vi "VerticalSpeedIndicator.vi"(6 "SignalSource":T1(ring), 7 "ScaleUnit(F=m/s; T=Ft/min/100)":bool=TRUE, 8 "error in (no error)":errorcluster caption="Fehler (Eingang, kein Fehler)", 10 "MultiWii Data Cluster":T2 {"Altitude abs [m]" format="%.2f"; "Baro T [°C]" format="%.1f"; "Baro P [mbara]" format="%.1f"; "GPS_coord[LON]" format="%#_9f"; "GPS_coord[LAT]" format="%#_9f"; "Altitude [m]" format="%.2f"}) -> (0 "error out":errorcluster caption="Fehler (Ausgang)", 2 "VerticalSpeedDigital":dbl format="%.1f", 3 "VerticalSpeedIndicator":picture)   [LabVIEW 2017]
uses:
  IMU_Functions/IMU_Data_Cluster.ctl
  <vilib>/picture/picture.llb/imagedata.ctl
  <vilib>/Utility/miscctls.llb/LVBoundsTypeDef.ctl
panel:
  in  "Transparent":picture caption="Neue Grafik"
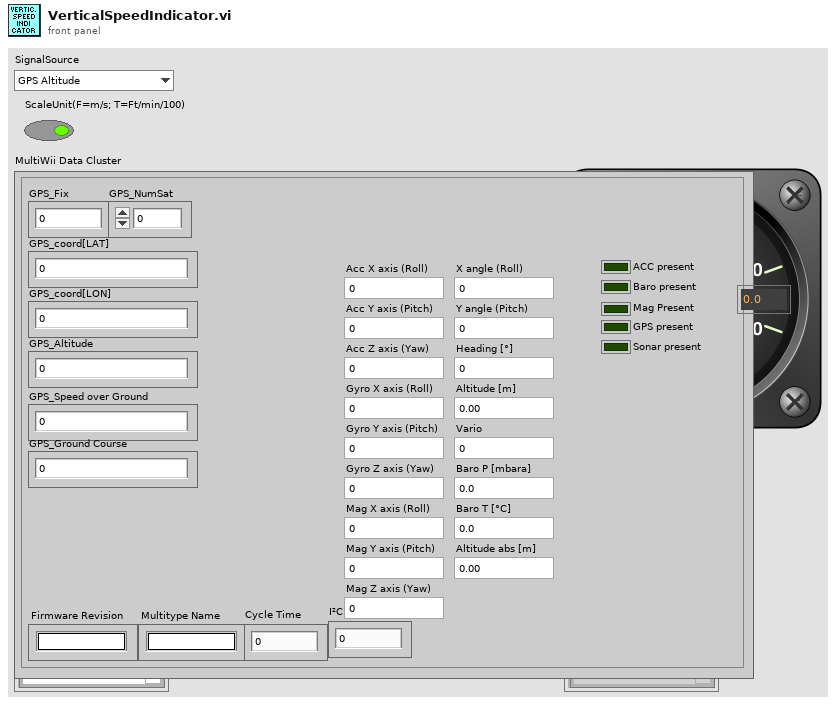
[diagram p1: front panel]
types:
  T1 = enum16{"GPS Altitude", "Baro absolute Altitude", "Baro Vario"}
  T2 = typedef "IMU_Data_Cluster.ctl" = cluster{"Firmware Revision":string, "Multitype Name":string, "Cycle Time":u16, "I²C Error Count":u16, "ACC present":bool, "Baro present":bool, "Mag Present":bool, "GPS present":bool, "Sonar present":bool, "Acc X axis (Roll)":dbl, "Acc Y axis (Pitch)":dbl, "Acc Z axis (Yaw)":dbl, "Gyro X axis (Roll)":dbl, "Gyro Y axis (Pitch)":dbl, "Gyro Z axis (Yaw)":dbl, "Mag X axis (Roll)":dbl, "Mag Y axis (Pitch)":dbl, "Mag Z axis (Yaw)":dbl, "X angle (Roll)":dbl, "Y angle (Pitch)":dbl, "Heading [°]":dbl, "Altitude [m]":dbl, "Vario":dbl, "GPS_Fix":u8, "GPS_NumSat":u8, "GPS_coord[LAT]":dbl, "GPS_coord[LON]":dbl, "GPS_Altitude":dbl, "GPS_Speed over Ground":dbl, "GPS_Ground Course":dbl, "Baro P [mbara]":dbl, "Baro T [°C]":dbl, "Altitude abs [m]":dbl}
  T3 = typedef "LVBoundsTypeDef.ctl" = cluster{"Width":u32, "Height":u32}
  T4 = typedef "imagedata.ctl" = cluster{"image type":i32, "image depth":i32, "image":u8[], "mask":u8[], "colors":u32[], "Rectangle":cluster{"left":i16, "top":i16, "right":i16, "bottom":i16}}
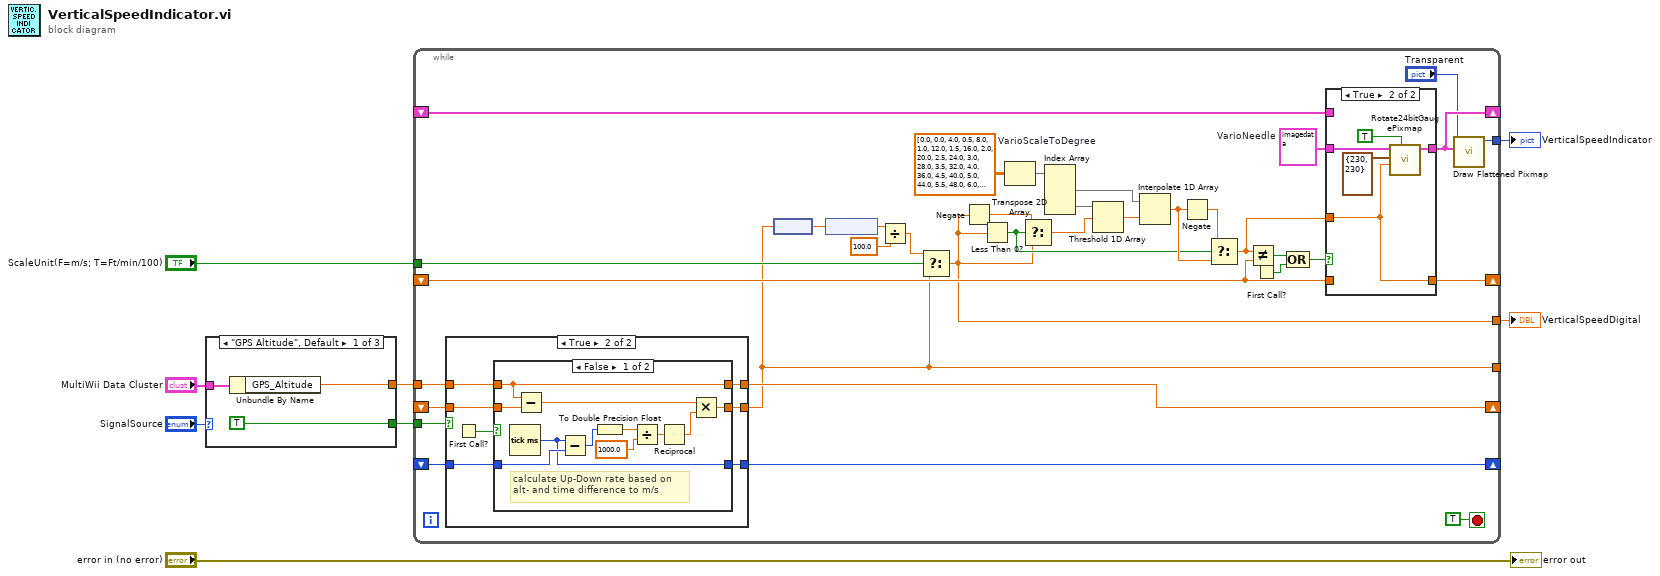
[diagram p0: block diagram]
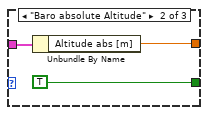
[diagram p2: hidden frame]
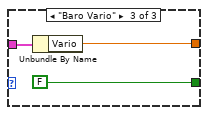
[diagram p3: hidden frame]
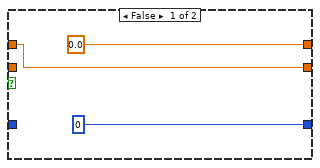
[diagram p4: hidden frame]
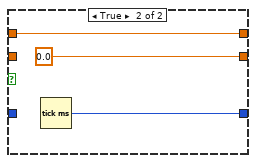
[diagram p5: hidden frame]
diagram:
  n1 = case shown="\"GPS Altitude\", Default" "SignalSource" {
    tunnel: [TRUE TRUE FALSE] -> w2
    tunnel: "MultiWii Data Cluster" -> [w11 w14 w16]
    tunnel: [w10 w12 w15] -> w3
    frame "GPS Altitude", Default {
      n2 = Unbundle By Name(w11) -> ("GPS_Altitude"=w10:dbl)
    }
    frame "Baro absolute Altitude" {
      n3 = Unbundle By Name(w14) -> ("Altitude abs [m]"=w12:dbl)
    }
    frame "Baro Vario" {
      n4 = Unbundle By Name(w16) -> ("Vario"=w15:dbl)
    }
  }
  n5 = while {
    shift-right: [w50] -> _
    shift-left: _ -> [w44]
    shift-right: [w49] -> _
    shift-left: _ -> [w48]
    tunnel: [w46] -> w8
    tunnel: w3 -> [w23]
    tunnel: "ScaleUnit(F=m/s; T=Ft/min/100)" -> [w31]
    tunnel: [w18] -> w1
    tunnel: [w22] -> _
    shift-right: [w26] -> _
    shift-left: _ -> [w27]
    tunnel: w2 -> [w24]
    shift-right: [w21] -> _
    shift-left: _ -> [w20]
    stop <- TRUE stop-if-true
    w42 = dbl[][] [[0.0, 0.0], [4.0, 0.5], [8.0, 1.0], [12.0, 1.5], [16.0, 2.0], [20.0, 2.5], [24.0, 3.0], [28.0, 3.5], [32.0, 4.0], [36.0, 4.5], [40.0, 5.0], [44.0, 5.5], [48.0, 6.0], [52.0, 6.5], [56.0, 7.0], [60.0, 7.5], [64.0, 8.0], [68.0, 8.5], [72.0, 9.0], [76.0, 9.5], [80.0, 10.0], [88.0, 11.0], [96.0, 12.0], [104.0, 13.0], [112.0, 14.0], [120.0, 15.0], [128.0, 16.0], [136.0, 17.0], [144.0, 18.0], [152.0, 19.0], [160.0, 20.0]]  # VarioScaleToDegree
    w43 = T4 {"image type"=0, "image depth"=24, "image"=array[158700 elements], "mask"=[], "colors"=[], "Rectangle"={"left"=0, "top"=0, "right"=230, "bottom"=230}}  # VarioNeedle
    n6 = case shown="True" w24 {
      tunnel: w27 -> [_ w62]
      tunnel: [0.0 ("VerticalSpeed (m/s)") w61] -> w26
      tunnel: w23 -> [w54 w60]
      tunnel: [w54 w58] -> w22
      tunnel: [u32 0 ("millisecond timer value") w57] -> w21
      tunnel: w20 -> [_ w56]
      frame False {
      }
      frame True {
        n7 = First Call?() -> (First Call?: T/F=w59:bool)
        n8 = case shown="False" w59 {
          tunnel: w60 -> [w72 w76]
          tunnel: [w72 w76] -> w61
          tunnel: w62 -> [w73 _]
          tunnel: [w65 0.0] -> w58
          tunnel: [w70 w74] -> w57
          tunnel: w56 -> [w71 _]
          frame False {
            # "calculate Up-Down rate based on\nalt- and time difference to m/s"
            n9 = Tick Count (ms)() -> (millisecond timer value=w70:u32)
            n10 = Subtract(x=w72, y=w73) -> (x-y=w64:dbl)
            n11 = Subtract(x=w70, y=w71) -> (x-y=w69:u32)
            n12 = To Double Precision Float(number=w69) -> (double precision float=w68:dbl)
            n13 = Divide(x=w68, y=1000.0) -> (x/y=w66:dbl)
            n14 = Reciprocal(x=w66) -> (1/x=w63:dbl)
            n15 = Multiply(x=w64, y=w63) -> (x*y=w65:dbl)
          }
          frame True {
            n16 = Tick Count (ms)() -> (millisecond timer value=w74:u32)
          }
        }
      }
    }
    n17 = node(w22) -> (w30:dbl[unit])
    n18 = node(w30) -> (w29:dbl)
    n19 = Divide(x=w29, y=100.0) -> (x/y=w19:dbl)
    n20 = Select(t=w19, s=w31, f=w22) -> (s? t:f=w18:dbl)
    n21 = Negate(x=w18) -> (-x=w37:dbl)
    n22 = Less Than 0?(x=w18) -> (x < 0?=w39:bool)
    n23 = Transpose 2D Array(2D array=w42) -> (transposed array=w34:dbl[][])
    n24 = Select(t=w37, s=w39, f=w18) -> (s? t:f=w38:dbl)
    n25 = Index Array(array=w34) -> (element #1=w36:dbl[], element #2=w35:dbl[])  [unwired: 4 in]
    n26 = Threshold 1D Array(2:w38, 3:w35) -> (0:w33:dbl)  [unwired: 1 in]
    n27 = Interpolate 1D Array(1:w33, 2:w36) -> (0:w41:dbl)
    n28 = Negate(x=w41) -> (-x=w40:dbl)
    n29 = Select(t=w40, s=w39, f=w41) -> (s? t:f=w32:dbl)
    n30 = Not Equal?(x=w32, y=w44) -> (x != y?=w51:bool)
    n31 = First Call?() -> (First Call?: T/F=w25:bool)
    n32 = Compound Arithmetic op=OR(w51, w25) -> (w52:bool)
    n33 = case shown="True" w52 {
      tunnel: w43 -> [_ w83]
      tunnel: [w78 w82] -> w49
      tunnel: w48 -> [w78 _]
      tunnel: w44 -> [w77 _]
      tunnel: [w77 w80] -> w50
      tunnel: w32 -> [_ w80]
      frame False {
      }
      frame True {
        n34 = call "Rotate24bitGaugePixmap.vi"("Maske kombinieren? (F)"=TRUE, "Rotation Angle (degrees)"=w80, "Größe des Darstellungsbereichs"=T3 {"Width"=230, "Height"=230}, "image data"=w83) -> ("image data out"=w82:T4)  [unwired: 7 in]
      }
    }
    n35 = call <vilib>:"Draw Flattened Pixmap.vi"("image data"=w49, "picture"="Transparent") -> ("new picture"=w46:picture)  [unwired: 7 out]
  }
  "VerticalSpeedIndicator" <- w8
  "VerticalSpeedDigital" <- w1
  "error out" <- "error in (no error)"
